vi "DefineJoint.vi"(0 "String 2":string, 2 "String":string) -> (4 "String 3":string)   [LabVIEW 2010]
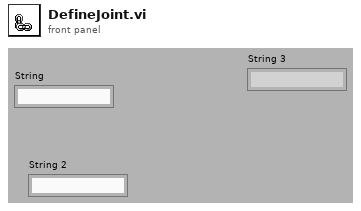
[diagram p1: front panel]
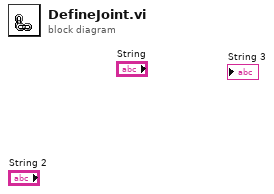
[diagram p0: block diagram]
diagram:
